vi "Dialog Example.vi"(4 "Python Message ID":i32, 5 "Script ID":i64, 7 "Server Alias":string, 8 "Error In":errorcluster, 10 "If Message Return Immediately":bool, 11 "Choices":string[](array[string])) -> (0 "Error Out":errorcluster, 3 "Choice":string)   [LabVIEW 2013]
doc: "This is an example of a dialog box for TestScript. The Python side can tell this dialog to run, asking for user input."
uses:
  LabVIEW Core/TS.lvlib
panel:
  out "Message":string
  in  "OK":bool
  in  "Choices":u16(ring) items=["Test complete!"]
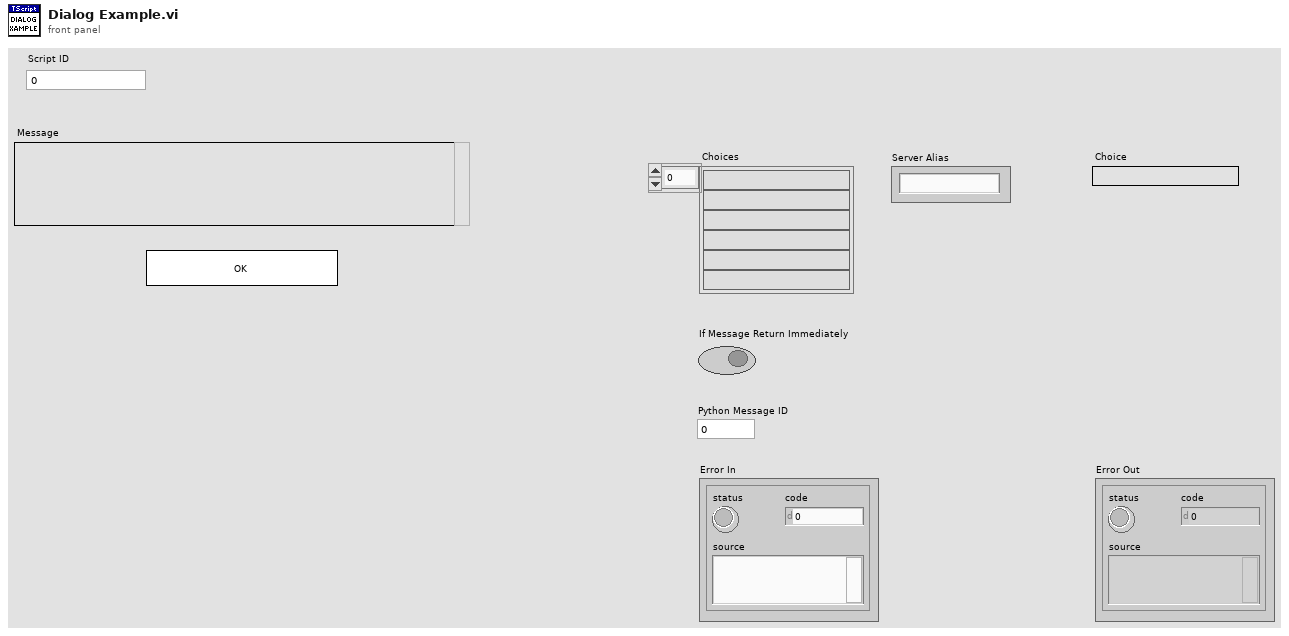
[diagram p1: front panel]
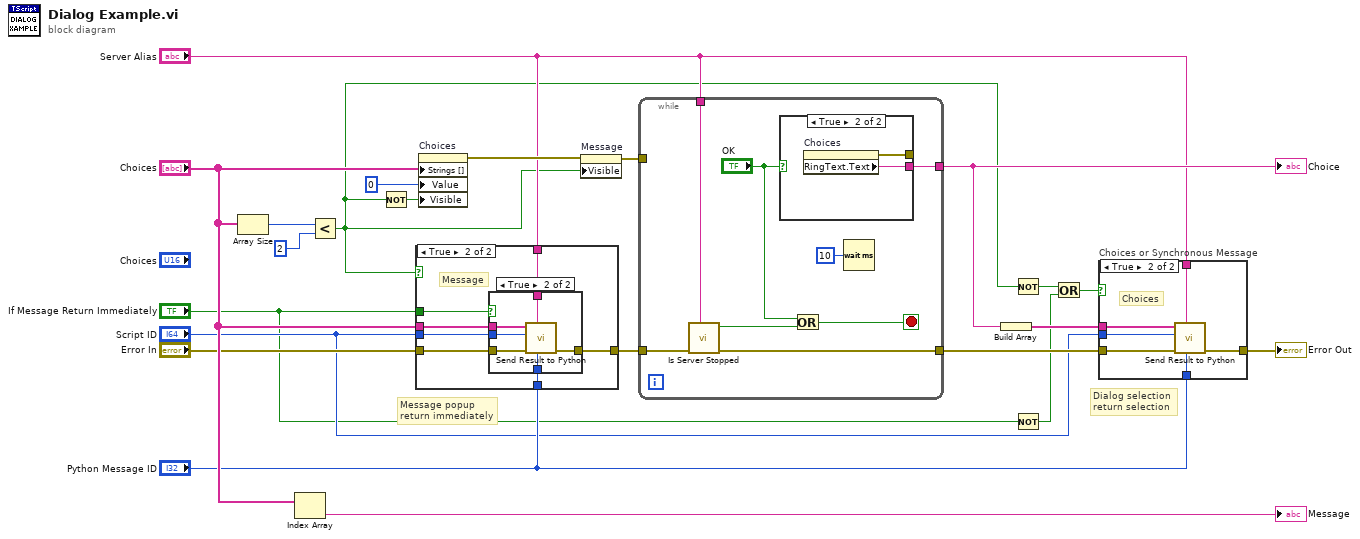
[diagram p0: block diagram]
diagram:
  # "Dialog selection\nreturn selection"
  # "Message popup\nreturn immediately"
  n1 = Array Size(array="Choices") -> (size(s)=w20:i32)
  n2 = Index Array(array="Choices") -> (element=→"Message":string)  [unwired: 1 in]
  n3 = Less?(x=w20, y=2) -> (x < y?=w5:bool)
  n4 = Not(x=w5) -> (.not. x?=w18:bool)
  n5 = case shown="True" w5 {
    tunnel: "Script ID" -> [_ w30]
    tunnel: "Choices" -> [_ w29]
    tunnel: "Python Message ID" -> [_ w28]
    tunnel: "Server Alias" -> [_ w27]
    tunnel: "Error In" -> [w23 w26]
    tunnel: [w23 w25] -> w9
    tunnel: "If Message Return Immediately" -> [_ w24]
    frame False {
      # "Choices"
      # "Choices"
    }
    frame True {
      # "Message"
      n6 = case shown="True" w24 {
        tunnel: w30 -> [_ w37]
        tunnel: w29 -> [_ w36]
        tunnel: w28 -> [_ w35]
        tunnel: w27 -> [_ w34]
        tunnel: w26 -> [w31 w33]
        tunnel: [w31 w32] -> w25
        frame False {
        }
        frame True {
          n7 = call "Send Result to Python.vi"("Python Message ID"=w35, "Server Alias"=w34, "error in (no error)"=w33, "Script ID"=w37, "Result Data"=w36) -> ("error out"=w32:errorcluster)  [unwired: 6 in]
        }
      }
    }
  }
  n8 = property on="Choices" class="Ring (strict)"("Strings []"="Choices", "Value"=u16 0 ("milliseconds to wait"), "Visible"=w18) -> (error out=w17:errorcluster)  [unwired: 2 in, 1 out]
  n9 = property on="Message" class="Str"(error in=w17, "Visible"=w5) -> (error out=w12:errorcluster)  [unwired: 1 in, 1 out]
  n10 = while {
    tunnel: [w44] -> w16
    tunnel: w12 -> [_]
    tunnel: w9 -> [w43]
    tunnel: [w42] -> w8
    tunnel: "Server Alias" -> [w41]
    stop <- w38 stop-if-true
    n11 = call "Is Server Stopped.vi"("Server Alias"=w41, "Error In"=w43) -> ("Error Out"=w42:errorcluster, "Server Stopped"=w40:bool)  [unwired: 8 in]
    n12 = case shown="True" "OK" {
      tunnel: [_ w47] -> w44
      tunnel: [_ w46] -> _
      frame False {
      }
      frame True {
        n13 = property on="Choices" class="Ring (strict)"() -> (error out=w46:errorcluster, "RingText.Text"=w47:string)  [unwired: 2 in, 1 out]
      }
    }
    n14 = Or(x="OK", y=w40) -> (x .or. y?=w38:bool)
    n15 = Wait (ms)(milliseconds to wait=u32 10) -> ()  [unwired: 1 out]
  }
  "Choice" <- w16
  n16 = Build Array(w16) -> (w14:string[])
  n17 = Not(x=w5) -> (.not. x?=w2:bool)
  n18 = Not(x="If Message Return Immediately") -> (.not. x?=w3:bool)
  n19 = Or(x=w2, y=w3) -> (x .or. y?=w1:bool)
  n20 = case "Choices or Synchronous Message" shown="True" w1 {
    tunnel: w14 -> [_ w54]
    tunnel: "Python Message ID" -> [_ w53]
    tunnel: "Server Alias" -> [_ w52]
    tunnel: w8 -> [w48 w51]
    tunnel: [w48 w50] -> w10
    tunnel: "Script ID" -> [_ w49]
    frame False {
      # "Message"
    }
    frame True {
      # "Choices"
      n21 = call "Send Result to Python.vi"("Python Message ID"=w53, "Server Alias"=w52, "error in (no error)"=w51, "Script ID"=w49, "Result Data"=w54) -> ("error out"=w50:errorcluster)  [unwired: 6 in]
    }
  }
  "Error Out" <- w10
